vi "SAE refroidisement 1.1.vi"() -> ()   [LabVIEW 2022 SP3]
uses:
  <vilib>/Analysis/baseanly.llb/Mean (DBL).vi
  <vilib>/Analysis/NI_AALBase.lvlib
panel:
  out "Tableau":dbl[](array[numeric])
  out "Temps":dbl
  out "Temperature":dbl
  out "Niveaux Temp  reel  2":dbl(graph)
  out "Chronos":dbl(knob) scale=0.0..100.0
  out "Thermometer 0-100":dbl(slide) scale=0.0..100.0
  out "Thermometer 20-30":dbl(slide) scale=20.0..29.0
  out "Moyenne":dbl format="%0.2f"
  out "Niveaux 1":bool
  out "Niveaux 2":bool
  out "Niveaux 3":bool
  out "XY Graph":cluster{dbl[], dbl[]}(graph)
  out "XY Graph 2":cluster{dbl[], dbl[]}(graph)
  out "Niveaux reel":i32(graph)
  in  "Seuil d'alerte":cluster{"Seuil B":dbl, "Seuil H":dbl}
  in  "stop (F)":bool
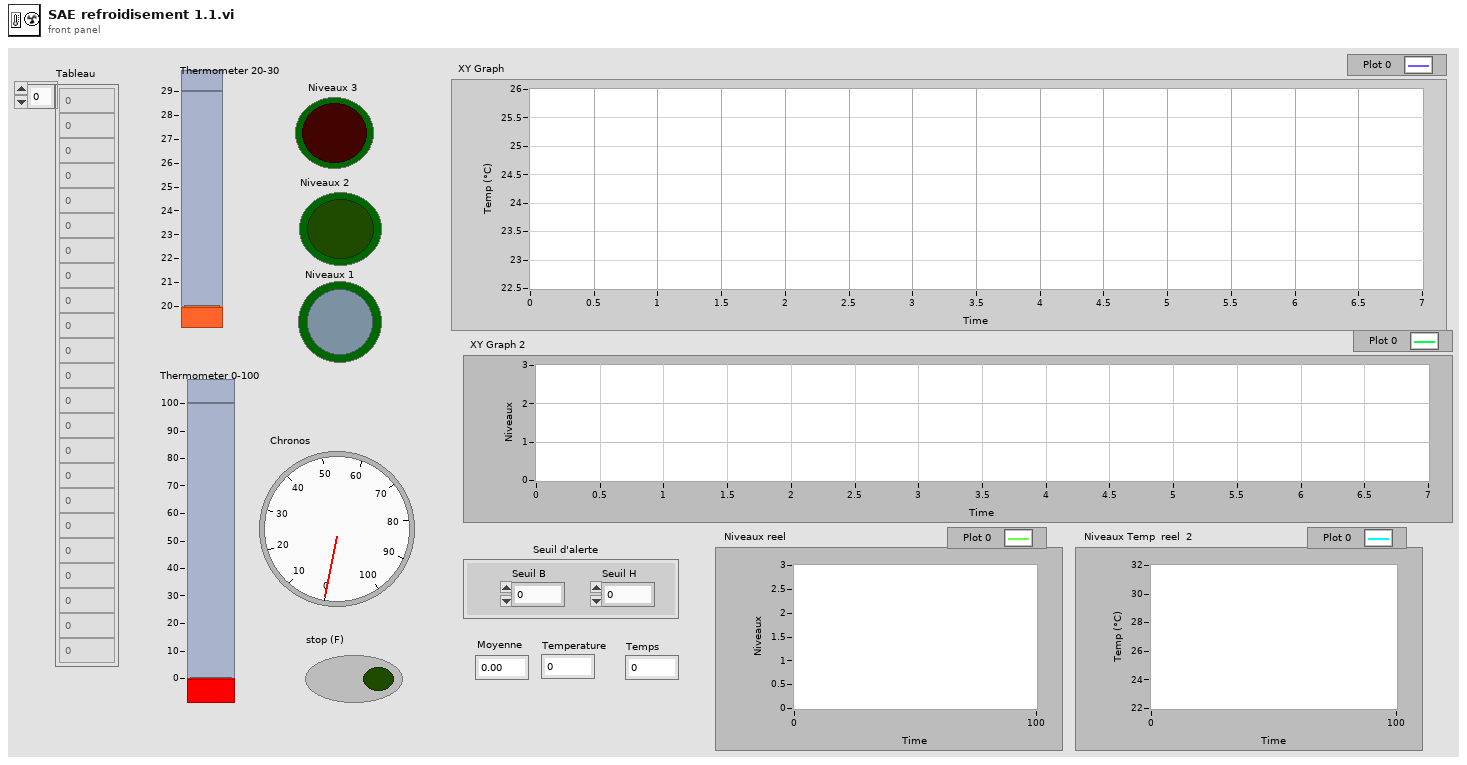
[diagram p1: front panel]
types:
  T1 = enum16{"open", "replace", "create", "open or create", "replace or create", "replace or create with confirmation"}
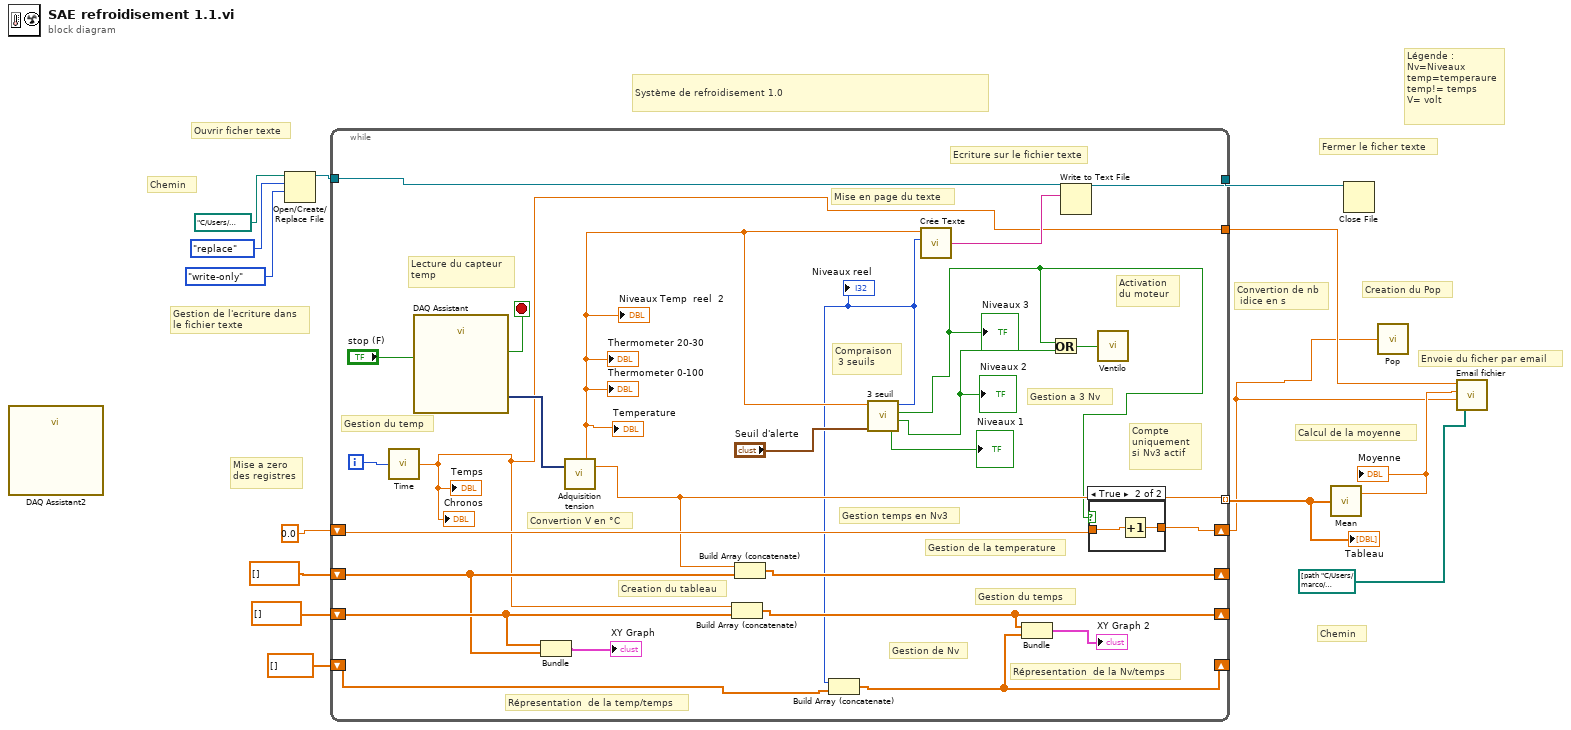
[diagram p0: block diagram]
diagram:
  # "Convertion de nb\n idice en s"
  # "Gestion de l'ecriture dans \nle fichier texte"
  # "Chemin"
  # "Chemin"
  # "Mise a zero \ndes registres"
  # "Calcul de la moyenne"
  # "Creation du Pop"
  # "Envoie du ficher par email"
  # "Légende :\nNv=Niveaux\ntemp=temperaure\ntemp!= temps\nV= volt"
  # "Système de refroidisement 1.0"
  # "Fermer le ficher texte"
  # "Ouvrir ficher texte"
  n1 = call "DAQ Assistant2"() -> ()  [unwired: 18 in, 2 out]
  n2 = Open/Create/Replace File(file path (use dialog)=path "C:/Users/marco/Documents/Ivan/IUT/SAE/Refroidisement labview/Resulta_texte.txt", operation (0:open)=T1."replace", access (0:read/write)=enum16{"read/write", "read-only", "write-only"}."write-only") -> (refnum out=w8:refnum<file>)  [unwired: 3 in, 2 out]
  n3 = while {
    tunnel: [w18] -> w5 mode=indexing
    shift-right: [w23] -> _
    shift-left: dbl[] [] -> [w35]
    shift-right: [w36] -> _
    shift-left: dbl[] [] -> [w34]
    shift-right: [w33] -> w1
    shift-left: 0.0 -> [w26]
    tunnel: w8 -> [w29]
    tunnel: [w30] -> w7
    shift-right: [w24] -> _
    shift-left: dbl[] [] -> [w25]
    tunnel: [w15] -> w4
    i -> [w31]
    stop <- w38 stop-if-true
    # "Ecriture sur le fichier texte"
    # "Compte \nuniquement \nsi Nv3 actif"
    # "Creation du tableau"
    # "Activation \ndu moteur"
    # "Gestion a 3 Nv"
    # "Compraison\n 3 seuils"
    # "Répresentation  de la Nv/temps"
    # "Répresentation  de la temp/temps"
    # "Gestion de Nv"
    # "Gestion du temps"
    # "Gestion de la temperature"
    # "Gestion temps en Nv3"
    # "Convertion V en °C"
    # "Gestion du temp"
    # "Mise en page du texte"
    # "Lecture du capteur \ntemp"
    n4 = call "Time.vi"("Indice"=w31) -> ("Temps (s)"=w15:dbl)
    "Chronos" <- w15
    "Temps" <- w15
    n5 = call "DAQ Assistant"("stop (F)"="stop (F)") -> ("data"=w37:dynamicdata, "stopped"=w38:bool)  [unwired: 15 in, 2 out]
    n6 = Bundle(w35, w34) -> (→"XY Graph":cluster{dbl[], dbl[]})  [unwired: 1 in]
    n7 = call "Adquisition tension.vi"("Tension"=w37) -> ("Température"=w18:dbl)  [unwired: 2 in]
    "Thermometer 20-30" <- w18
    "Thermometer 0-100" <- w18
    "Niveaux Temp  reel  2" <- w18
    "Temperature" <- w18
    n8 = Build Array (concatenate)(w15, w35) -> (w23:dbl[])
    n9 = Build Array (concatenate)(w18, w34) -> (w36:dbl[])
    n10 = call "3 seuil.vi"("Seuil"="Seuil d'alerte", "Temp"=w18) -> ("Niveaux 1"=→"Niveaux 1":bool, "Niveaux 2"=w19:bool, "Niveaux 3"=w16:bool, "Niveaux"=w17:i32)  [unwired: 2 in]
    "Niveaux reel" <- w17
    "Niveaux 3" <- w16
    "Niveaux 2" <- w19
    n11 = Build Array (concatenate)(w17, w25) -> (w24:dbl[])
    n12 = call "Crée Texte.vi"("Niveaux"=w17, "Temperature"=w18) -> ("Texte"=w28:string)  [unwired: 2 in]
    n13 = Bundle(w23, w24) -> (→"XY Graph 2":cluster{dbl[], dbl[]})  [unwired: 1 in]
    n14 = Or(x=w16, y=w19) -> (x .or. y?=w32:bool)
    n15 = Write to Text File(file (use dialog)=w29, text=w28) -> (refnum out=w30:refnum<file>)  [unwired: 2 in, 2 out]
    n16 = case shown="True" w16 {
      tunnel: [w40 w42] -> w33
      tunnel: w26 -> [w40 w41]
      frame False {
      }
      frame True {
        n17 = Increment(x=w41) -> (x+1=w42:dbl)
      }
    }
    n18 = call "Ventilo.vi"("Boolean"=w32) -> ()
  }
  "Tableau" <- w5
  n19 = call-poly <vilib>:"Mean.vi"("X"=w5) -> ("mean"=w2:dbl)  [unwired: 1 out]
  "Moyenne" <- w2
  n20 = Close File(refnum=w7) -> ()  [unwired: 1 in, 2 out]
  n21 = call "Pop.vi"("nb idice nv3"=w1) -> ()
  n22 = call "Email fichier.vi"("attachments"=path[] [path "C:/Users/marco/Documents/Ivan/IUT/SAE/Refroidisement labview/Resulta_texte.txt"], "nb idice nv3"=w1, "moyenne"=w2, "Temp exp"=w4) -> ()  [unwired: 1 in]
